vi "session_callback_send.vi"(8 "error in (no error)":errorcluster, 9 "flags":i32, 10 "buffer":u8[](array[numeric]), 11 "socket":u64) -> (0 "error out":errorcluster, 2 "bytes send":i64)   [LabVIEW 2017]
doc: "Called when libssh2 wants to send data on the connection.\n\n<B>socket</B> is the socket to write to.\n<B>buffer</B> is the data to send.\n<B>flags</B> are the flags that would have been used by a send() call.\n\nReturns the number of bytes sent."
uses:
  ws2_32.dll
  libc.so.6
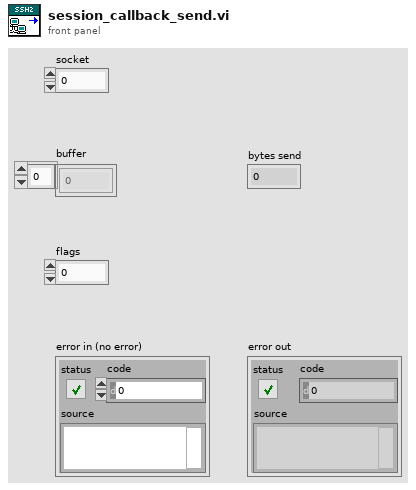
[diagram p1: front panel]
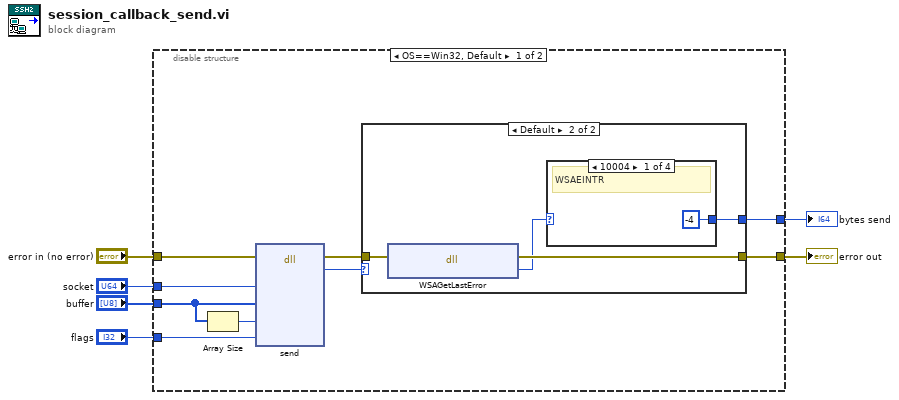
[diagram p0: block diagram]
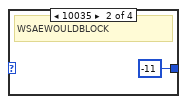
[diagram p3: hidden frame]
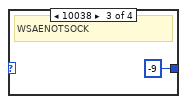
[diagram p4: hidden frame]
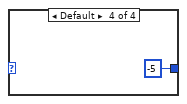
[diagram p5: hidden frame]
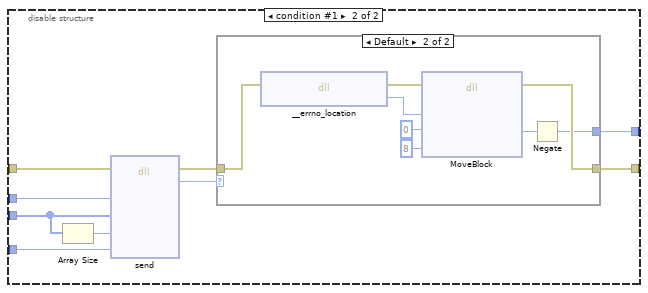
[diagram p6: hidden frame]
diagram:
  n1 = disable-structure shown="OS==Win32, Default" {
    disable-tunnel: "error in (no error)" -> [w15 w34]
    disable-tunnel: "socket" -> [w14 w33]
    disable-tunnel: "buffer" -> [w12 w32]
    disable-tunnel: "flags" -> [w11 w30]
    disable-tunnel: [w8 w26] -> w2
    disable-tunnel: [w7 w28] -> w1
    frame condition #0 (active) {
      n2 = Array Size(array=w12) -> (size(s)=w13:i32)
      n3 = dll-call lib="ws2_32.dll" fn="send"(error in=w15, "s"=w14, "buf"=w12, "len"=w13, "flags"=w11) -> (error out=w10:errorcluster, "return type"=w9:i32)  [unwired: 6 in, 1 out]
      n4 = case shown="Default" w9 {
        selector: w9 -> [w17 _]
        tunnel: w10 -> [w16 w21]
        tunnel: [w16 w20] -> w7
        tunnel: [w17 w18] -> w8
        frame 0.. {
        }
        frame Default {
          n5 = dll-call lib="ws2_32.dll" fn="WSAGetLastError"(error in=w21) -> (error out=w20:errorcluster, "return type"=w19:i32)  [unwired: 2 in, 1 out]
          n6 = case shown="10004" w19 {
            tunnel: [-4 -11 -9 -5] -> w18
            frame 10004 {
              # "WSAEINTR"
            }
            frame 10035 {
              # "WSAEWOULDBLOCK"
            }
            frame 10038 {
              # "WSAENOTSOCK"
            }
            frame Default {
            }
          }
        }
      }
    }
    frame condition #1 {
      n7 = Array Size(array=w32) -> (size(s)=w31:i32)
      n8 = dll-call lib="libc.so.6" fn="send"(error in=w34, "sockfd"=w33, "buf"=w32, "size"=w31, "flags"=w30) -> (error out=w29:errorcluster, "return type"=w27:i32)  [unwired: 6 in, 1 out]
      n9 = case shown="Default" w27 {
        selector: w27 -> [w36 _]
        tunnel: w29 -> [w35 w44]
        tunnel: [w35 w41] -> w28
        tunnel: [w36 w37] -> w26
        frame 0.. {
        }
        frame Default {
          n10 = dll-call lib="libc.so.6" fn="__errno_location"(error in=w44) -> (error out=w42:errorcluster, "return type"=w40:u64)  [unwired: 2 in, 1 out]
          n11 = dll-call lib="LabVIEW" fn="MoveBlock"(error in=w42, "ps"=w40, "pd"=0, "size"=u64 8) -> (error out=w41:errorcluster, "pd"=w38:i32)  [unwired: 5 in, 1 out]
          n12 = Negate(x=w38) -> (-x=w37:i32)
        }
      }
    }
  }
  "error out" <- w1
  "bytes send" <- w2
